vi "Serialize Host LLP Packets.vi"(0 "host llp packets":T2[](array[typedef]), 11 "error in (no error)":errorcluster) -> (4 "packet bytes":u8[](array[numeric]), 6 "packet sizes":u32[](array[numeric]), 8 "packet data types":T1[](array[typedef]), 15 "error out":errorcluster)   [LabVIEW 2023, in "GettingStarted_Gen_148X_Host.lvlib"]
uses:
  GettingStarted_Gen_148X_Host.lvlib
  <instrlib>/FlexRIO/CSI-2/v2/Host/Types/Host LLP Packet.ctl
  <instrlib>/FlexRIO/CSI-2/v2/FPGA/Types/LLP Packet Header.ctl
  <instrlib>/FlexRIO/CSI-2/v2/FPGA/Types/LLP Packet Footer.ctl
  <instrlib>/FlexRIO/CSI-2/v2/Common/Types/LLP Data Type.ctl
  <instrlib>/FlexRIO/CSI-2/v2/FPGA/NI CSI-2 API FPGA v2.lvlib
  <instrlib>/FlexRIO/CSI-2/v2/Common/NI CSI-2 API Common v2.lvlib
  <instrlib>/FlexRIO/CSI-2/v2/Host/NI CSI-2 API Host v2.lvlib
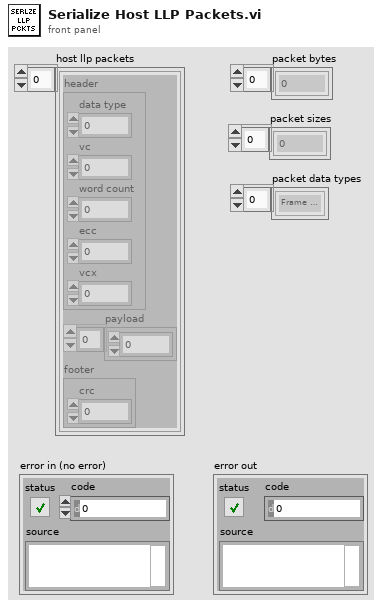
[diagram p1: front panel]
types:
  T1 = typedef "NI CSI-2 API Common v2.lvlib/LLP Data Type.ctl" = enum8{"Frame Start", "Frame End", "Line Start", "Line End", "End of Transmission", "Reserved 0", "Reserved 1", "Reserved 2", "Generic Short Packet 1", "Generic Short Packet 2", "Generic Short Packet 3", "Generic Short Packet 4", "Generic Short Packet 5", "Generic Short Packet 6", "Generic Short Packet 7", "Generic Short Packet 8", "Null", "Blanking Data", "Embedded 8-bit non Image Data", "Generic Long Packet 1", "Generic Long Packet 2", "Generic Long Packet 3", "Generic Long Packet 4", "Reserved 3", "YUV420 8-bit", "YUV420 10-bit", "Legacy YUV420 8-bit", "Reserved 4", "YUV420 8-bit Chroma Shifted", "YUV420 10-bit Chroma Shifted", "YUV422 8-bit", "YUV422 10-bit", "RGB444", "RGB555", "RGB565", "RGB666", "RGB888", "Reserved 5", "Reserved 6", "RAW 24", "RAW 6", "RAW 7", "RAW 8", "RAW 10", "RAW 12", "RAW 14", "RAW 16", "RAW 20", "User Defined 8-bit Data 1", "User Defined 8-bit Data 2", "User Defined 8-bit Data 3", "User Defined 8-bit Data 4", "User Defined 8-bit Data 5", "User Defined 8-bit Data 6", "User Defined 8-bit Data 7", "User Defined 8-bit Data 8", "USL Command", "Reserved 7", "Reserved 8", "Reserved 9", "Reserved 10", "Reserved 11", "Reserved 12", "LRTE EPD Spacer"}
  T2 = typedef "NI CSI-2 API Host v2.lvlib/Host LLP Packet.ctl" = cluster{"header":T3, "payload":u8[], "footer":T4}
  T3 = typedef "NI CSI-2 API FPGA v2.lvlib/LLP Packet Header.ctl" = cluster{"word count":u16, "ecc":fxp<+,6,6>, "vcx":fxp<+,2,2>, "data type":fxp<+,6,6>, "vc":fxp<+,2,2>}
  T4 = typedef "NI CSI-2 API FPGA v2.lvlib/LLP Packet Footer.ctl" = cluster{"crc":u16}
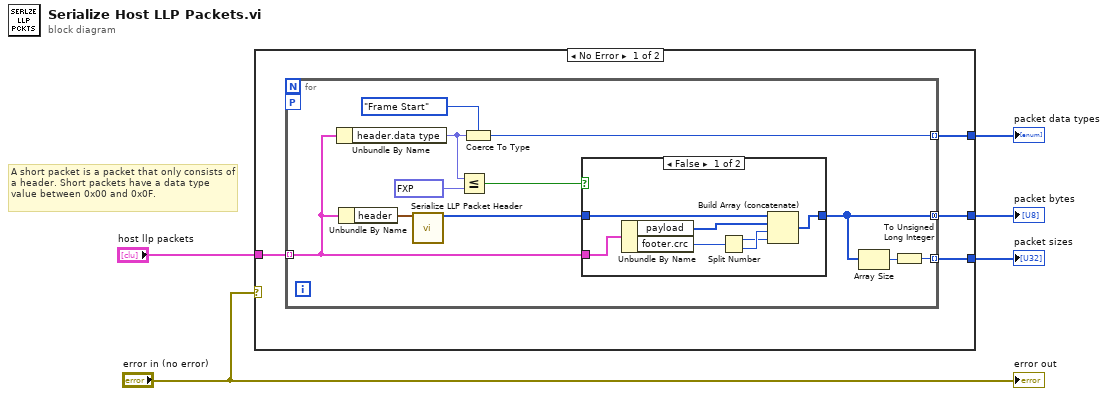
[diagram p0: block diagram]
diagram:
  # "A short packet is a packet that only consists of a header. Short packets have a data type value between 0x00 and 0x0F."
  n1 = case shown="No Error" "error in (no error)" {
    tunnel: [w9 _] -> w5
    tunnel: [w8 _] -> w4
    tunnel: "host llp packets" -> [w7 _]
    tunnel: [w6 _] -> w1
    frame No Error {
      n2 = for {
        tunnel: w7 -> [w15] mode=indexing
        tunnel: [w16] -> w8 mode=concatenating
        tunnel: [w20] -> w9 mode=indexing
        workers-P: _ -> [_]
        tunnel: [w13] -> w6 mode=indexing
        n3 = Unbundle By Name(w15) -> ("header.data type"=w11:fxp<+,6,6>)
        n4 = Unbundle By Name(w15) -> ("header"=w19:T3)
        n5 = call <instrlib>:"Serialize LLP Packet Header.vi"("header"=w19) -> ("serialized data"=w18:u8[])  [unwired: 14 in]
        n6 = Less Or Equal?(x=w11, y=fxp<+,6,6> 15.0 ("data type")) -> (x <= y?=w10:bool)
        n7 = Coerce To Type(0:w11, 1:LLP_Data_Type."Frame Start" ("Enum")) -> (2:w13:T1)
        n8 = case shown="False" w10 {
          tunnel: w18 -> [w25 w28]
          tunnel: [w27 w28] -> w16
          tunnel: w15 -> [w26 _]
          frame False {
            n9 = Unbundle By Name(w26) -> ("payload"=w24:u8[], "footer.crc"=w23:u16)
            n10 = Split Number(x=w23) -> (hi(x)=w21:u8, lo(x)=w22:u8)
            n11 = Build Array (concatenate)(w25, w24, w22, w21) -> (w27:u8[])
          }
          frame True {
          }
        }
        n12 = Array Size(array=w16) -> (size(s)=w17:i32)
        n13 = To Unsigned Long Integer(number=w17) -> (unsigned 32bit integer=w20:u32)
      }
    }
    frame Error {
    }
  }
  "packet sizes" <- w5
  "packet bytes" <- w4
  "packet data types" <- w1
  "error out" <- "error in (no error)"
